vi "Post_Dust_Event_Tick.vi"(7 "error in (no error)":errorcluster, 10 "Input Data":T1 {"Estimate Source" items=["Any Source."=-2, "No Shot"=-1, "Basic Labview Estimate"=0, "IDL Estimate From Andrew"=1, "IDL Estimate From Tobin"=2, "Old Metadata"=3]}) -> (0 "error out":errorcluster)   [LabVIEW 2013]
uses:
  Dust_Event.ctl
  Signal.ctl
  Private/Role ID.ctl
  Private/Hardware ID.ctl
  Private/Estimate_source.ctl
panel:
  # "Dust Event"
  # "Signal"
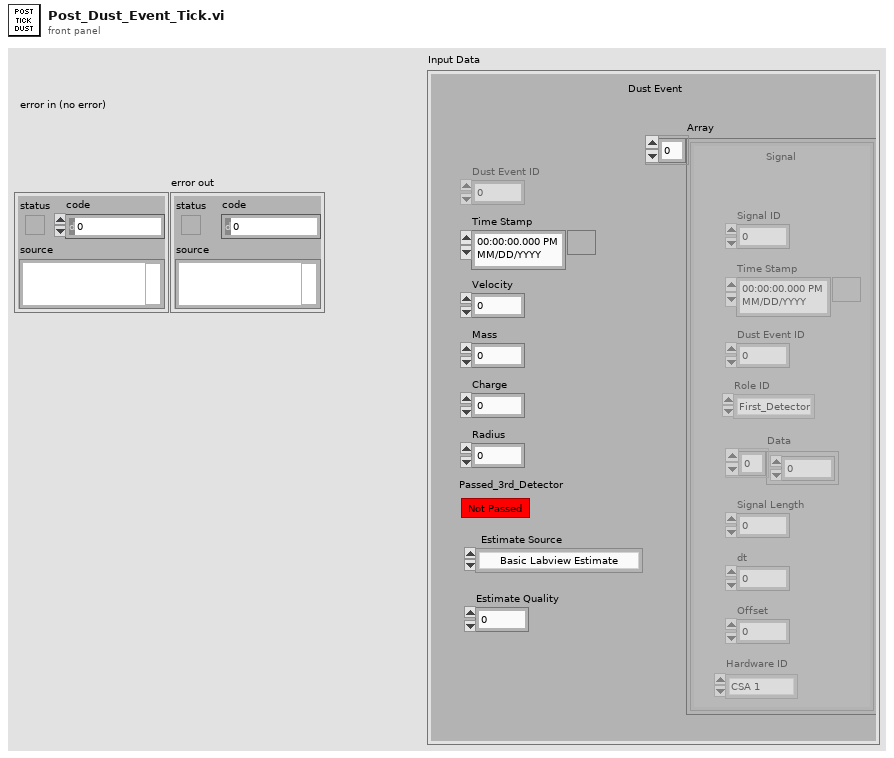
[diagram p1: front panel]
types:
  T1 = typedef "Dust_Event.ctl" = cluster{"Time Stamp":timestamp, "Velocity":sgl, "Mass":sgl, "Charge":sgl, "Radius":sgl, "Array":T2[], "Dust Event ID":i64, "Passed_3rd_Detector":bool, "Estimate Source":T5, "Estimate Quality":sgl}
  T2 = typedef "Signal.ctl" = cluster{"Signal ID":i64, "Time Stamp":timestamp, "Dust Event ID":i64, "Role ID":T3, "Data":sgl[], "Signal Length":i32, "dt":sgl, "Offset":dbl, "Hardware ID":T4}
  T3 = typedef "Role ID.ctl" = enum16{"First_Detector", "Second_Detector", "Third_Detector", "LeCroy_CH1", "LeCroy_CH2", "LeCroy_CH3", "LeCroy_CH4", "PSU"}
  T4 = typedef "Hardware ID.ctl" = enum16{"Unknown", "CSA 1", "CSA 2", "CSA 3", "CSA 4", "CSA 5", "CSA 6"}
  T5 = typedef "Estimate_source.ctl" = i8
  T6 = typedef "Semaphore RefNum" = refnum<k1>
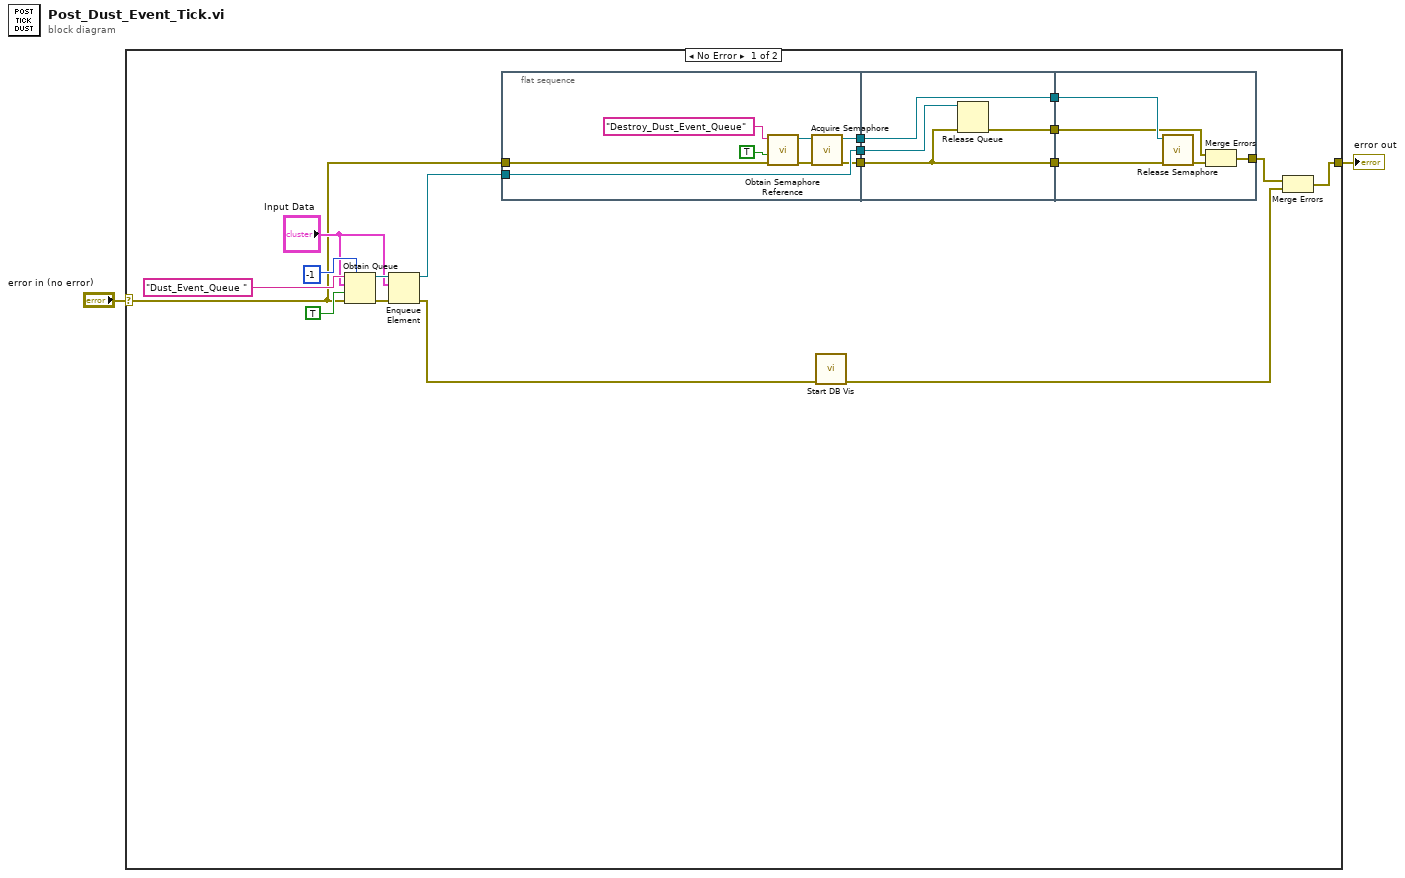
[diagram p0: block diagram]
diagram:
  n1 = case shown="No Error" "error in (no error)" {
    selector: "error in (no error)" -> [w13 w38]
    tunnel: [w5 w38] -> w1
    frame No Error {
      n2 = Obtain Queue(max queue size (-1, unlimited)=-1, name (unnamed)="Dust_Event_Queue ", element data type="Input Data", create if not found? (T)=TRUE, error in (no error)=w13) -> (queue out=w20:refnum<queue>, error out=w14:errorcluster)  [unwired: 1 out]
      n3 = Enqueue Element(queue=w20, element="Input Data", error in (no error)=w14) -> (queue out=w16:refnum<queue>, error out=w4:errorcluster)  [unwired: 1 in, 1 out]
      n4 = flat-sequence {
        tunnel: w13 -> [w23]
        tunnel: w16 -> [w28]
        tunnel: [w28] -> w12
        tunnel: [w22] -> w11
        tunnel: [w21] -> w9
        tunnel: w12 -> [w32]
        tunnel: w11 -> [w29]
        tunnel: [w31] -> w10
        tunnel: w9 -> [w30]
        tunnel: [w30] -> w8
        tunnel: [w29] -> w7
        tunnel: [w33] -> w6
        tunnel: w10 -> [w35]
        tunnel: w8 -> [w36]
        tunnel: w7 -> [w37]
        frame #0 {
          n5 = call <vilib>:"Obtain Semaphore Reference.vi"("error in (no error)"=w23, "create if not found (T)"=TRUE, "name (unnamed)"="Destroy_Dust_Event_Queue") -> ("error out"=w25:errorcluster, "semaphore"=w24:T6)  [unwired: 2 in, 1 out]
          n6 = call <vilib>:"Acquire Semaphore.vi"("error in (no error)"=w25, "semaphore"=w24) -> ("error out"=w22:errorcluster, "semaphore out"=w21:T6)  [unwired: 3 in, 1 out]
        }
        frame #1 {
          n7 = Release Queue(queue=w32, error in (no error)=w29) -> (error out=w31:errorcluster)  [unwired: 1 in, 2 out]
        }
        frame #2 {
          n8 = call <vilib>:"Release Semaphore.vi"("error in (no error)"=w37, "semaphore"=w36) -> ("error out"=w34:errorcluster)  [unwired: 4 in, 1 out]
          n9 = Merge Errors(w35, w34) -> (w33:errorcluster)
        }
      }
      n10 = call "Start DB Vis.vi"("error in (no error)"=w4) -> ("error out"=w3:errorcluster)  [unwired: 10 in]
      n11 = Merge Errors(w6, w3) -> (w5:errorcluster)
    }
    frame Error {
    }
  }
  "error out" <- w1
